vi "JakeInputIO.vi"() -> ()   [LabVIEW 2016]
uses:
  <vilib>/Analysis/baseanly.llb/Mean (DBL).vi
  <vilib>/measure/mamon.llb/Waveform Peak Detection for 1 Chan.vi
  <vilib>/Waveform/WDTOps.llb/WDT Append Waveforms DBL.vi
  <vilib>/measure/NI_MAPro.lvlib
  <vilib>/Analysis/NI_AALBase.lvlib
panel:
  out "Raw Audio\nWaveform":waveform(dbl)(graph)
  out "Amplitude Waveform":waveform(dbl)(graph)
  out "Waveform Chart":waveform(dbl)(graph)
  in  "stop (F)":bool
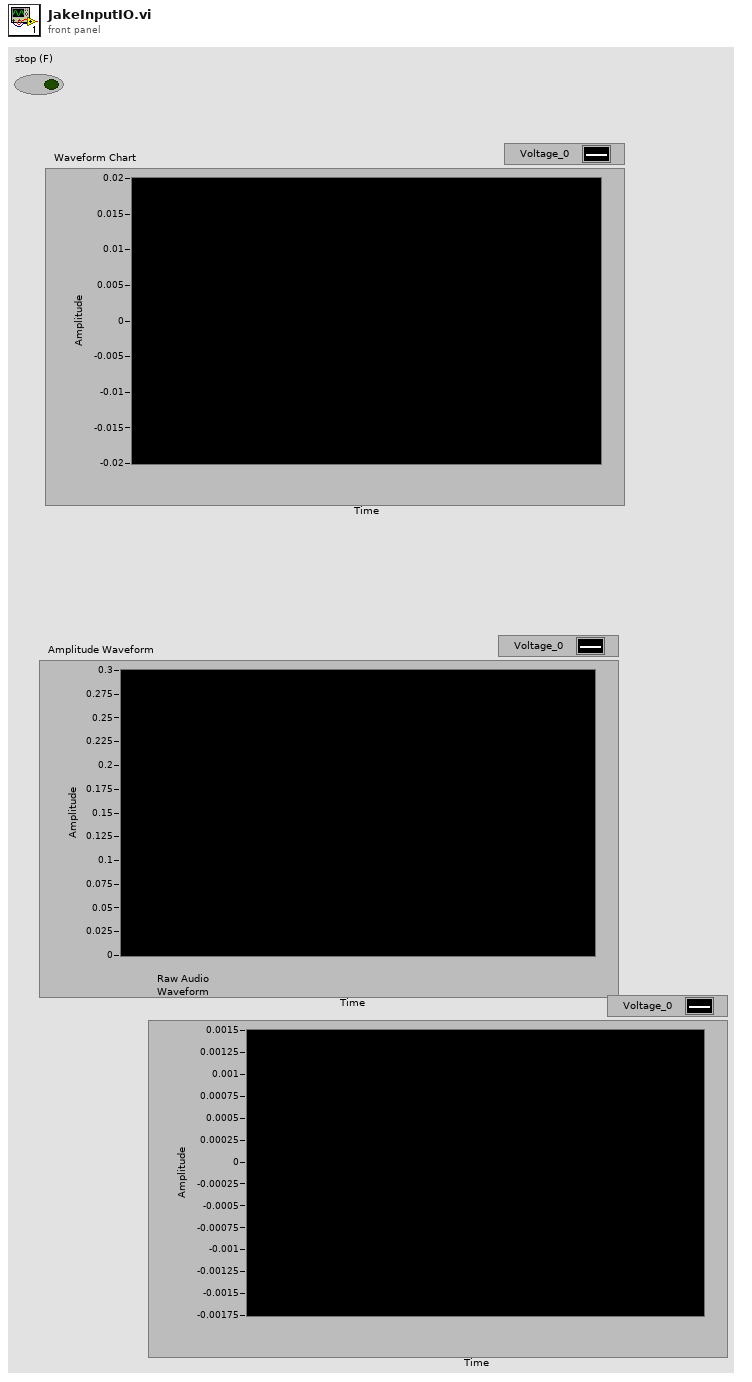
[diagram p1: front panel]
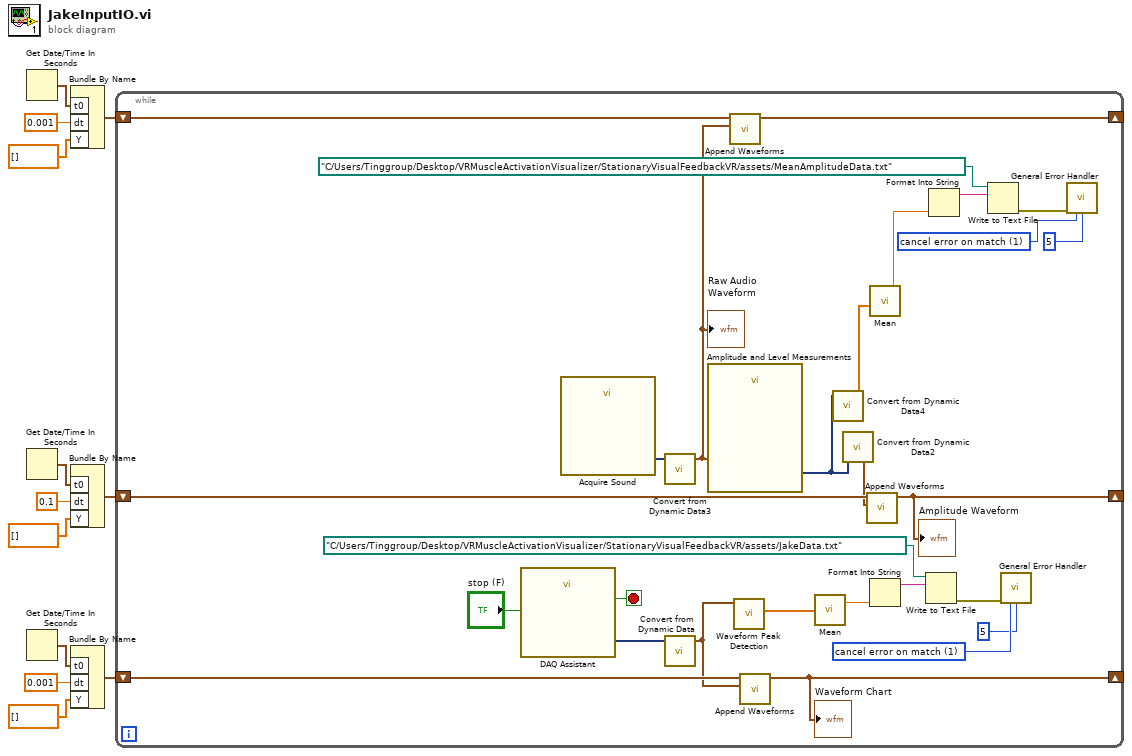
[diagram p0: block diagram]
diagram:
  n1 = Get Date/Time In Seconds() -> (seconds since 1Jan1904=w3:timestamp)
  n2 = Get Date/Time In Seconds() -> (seconds since 1Jan1904=w7:timestamp)
  n3 = Get Date/Time In Seconds() -> (seconds since 1Jan1904=w10:timestamp)
  n4 = Bundle By Name("t0"=w3, "dt"=0.001, "Y"=dbl[] []) -> (w1:waveform(dbl))  [unwired: 1 in]
  n5 = Bundle By Name("t0"=w7, "dt"=0.1, "Y"=dbl[] []) -> (w5:waveform(dbl))  [unwired: 1 in]
  n6 = Bundle By Name("t0"=w10, "dt"=0.001, "Y"=dbl[] []) -> (w12:waveform(dbl))  [unwired: 1 in]
  n7 = while {
    shift-right: [w36] -> _
    shift-left: w12 -> [w37]
    shift-right: [w27] -> _
    shift-left: w5 -> [w28]
    shift-right: [w23] -> _
    shift-left: w1 -> [w24]
    stop <- w39 stop-if-true
    w21 = 1 items=["no exception", "cancel error on match", "set error on match"] ("[exception action] (none:0)")
    w30 = 1 items=["no exception", "cancel error on match", "set error on match"] ("[exception action] (none:0)")
    n8 = call "DAQ Assistant"("stop (F)"="stop (F)") -> ("data"=w38:dynamicdata, "stopped"=w39:bool)  [unwired: 15 in, 2 out]
    n9 = call "Acquire Sound"() -> ("Data"=w26:dynamicdata)  [unwired: 18 in, 1 out]
    n10 = call "Convert from Dynamic Data3"("Dynamic Data Type"=w26) -> ("Waveform"=w25:waveform(dbl))  [unwired: 3 in]
    "Raw Audio\nWaveform" <- w25
    n11 = call "Convert from Dynamic Data"("Dynamic Data Type"=w38) -> ("Waveform"=w17:waveform(dbl))  [unwired: 3 in]
    n12 = call "Amplitude and Level Measurements"("Signals"=w25) -> ("Positive Peak"=w15:dynamicdata)  [unwired: 13 in, 1 out]
    n13 = call-poly <vilib>:"Append Waveforms.vi"("waveform B"=w25, "waveform A"=w24) -> ("waveform out"=w23:waveform(dbl))  [unwired: 8 in, 1 out]
    n14 = call-poly <vilib>:"Waveform Peak Detection.vi"("Signal In"=w17) -> ("Amplitudes"=w35:dbl[])  [unwired: 6 in, 4 out]
    n15 = call-poly <vilib>:"Append Waveforms.vi"("waveform B"=w17, "waveform A"=w37) -> ("waveform out"=w36:waveform(dbl))  [unwired: 8 in, 1 out]
    "Waveform Chart" <- w36
    n16 = call-poly <vilib>:"Mean.vi"("X"=w35) -> ("mean"=w34:dbl)  [unwired: 1 out]
    n17 = call "Convert from Dynamic Data4"("Dynamic Data Type"=w15) -> ("Array"=w14:dbl[])  [unwired: 3 in]
    n18 = call "Convert from Dynamic Data2"("Dynamic Data Type"=w15) -> ("Waveform"=w16:waveform(dbl))  [unwired: 3 in]
    n19 = call-poly <vilib>:"Append Waveforms.vi"("waveform B"=w16, "waveform A"=w28) -> ("waveform out"=w27:waveform(dbl))  [unwired: 8 in, 1 out]
    "Amplitude Waveform" <- w27
    n20 = call-poly <vilib>:"Mean.vi"("X"=w14) -> ("mean"=w13:dbl)  [unwired: 1 out]
    n21 = Format Into String(w34) -> (resulting string=w33:string)  [unwired: 3 in, 1 out]
    n22 = Write to Text File(file (use dialog)=path "C:/Users/Tinggroup/Desktop/VRMuscleActivationVisualizer/StationaryVisualFeedbackVR/assets/JakeData.txt", text=w33) -> (error out=w31:errorcluster)  [unwired: 2 in, 2 out]
    n23 = Format Into String(w13) -> (resulting string=w19:string)  [unwired: 3 in, 1 out]
    n24 = Write to Text File(file (use dialog)=path "C:/Users/Tinggroup/Desktop/VRMuscleActivationVisualizer/StationaryVisualFeedbackVR/assets/MeanAmplitudeData.txt", text=w19) -> (error out=w22:errorcluster)  [unwired: 2 in, 2 out]
    n25 = call <vilib>:"General Error Handler.vi"("error in (no error)"=w31, "[exception action] (none:0)"=w30, "[exception code]"=5) -> ()  [unwired: 8 in, 5 out]
    n26 = call <vilib>:"General Error Handler.vi"("error in (no error)"=w22, "[exception action] (none:0)"=w21, "[exception code]"=5) -> ()  [unwired: 8 in, 5 out]
  }
